vi "Call.vi"(6 "Error":errorcluster, 10 "PayloadCluster":T1 {"MetadataCluster"."AbsoluteTime" format="%<%x %.3X>T"}, 11 "Actor":refnum<class "Actor.lvclass">) -> (2 "PayloadCluster":T1 {"MetadataCluster"."AbsoluteTime" format="%<%x %.3X>T"}, 3 "Actor":refnum<class "Actor.lvclass">, 4 "Error":errorcluster)   [LabVIEW 2020, in "_Template.lvlib" / "{{Message}}.lvlib"]
uses:
  {{Message}}.lvlib
  Message/Message.lvclass
  jettl/jettl/jettl.lvlib
  jettl/jettl/Actor/Actor.lvclass
  jettl/jettl/LifecycleEnum.ctl
  jettl/jettl/TellOriginEnum.ctl
  jettl/jettl/MetadataCluster.ctl
  PayloadCluster.ctl
  jettl/jettl/CustomMetadata/CustomMetadata.lvclass
panel:
  # "This front panel should not be manipulated."
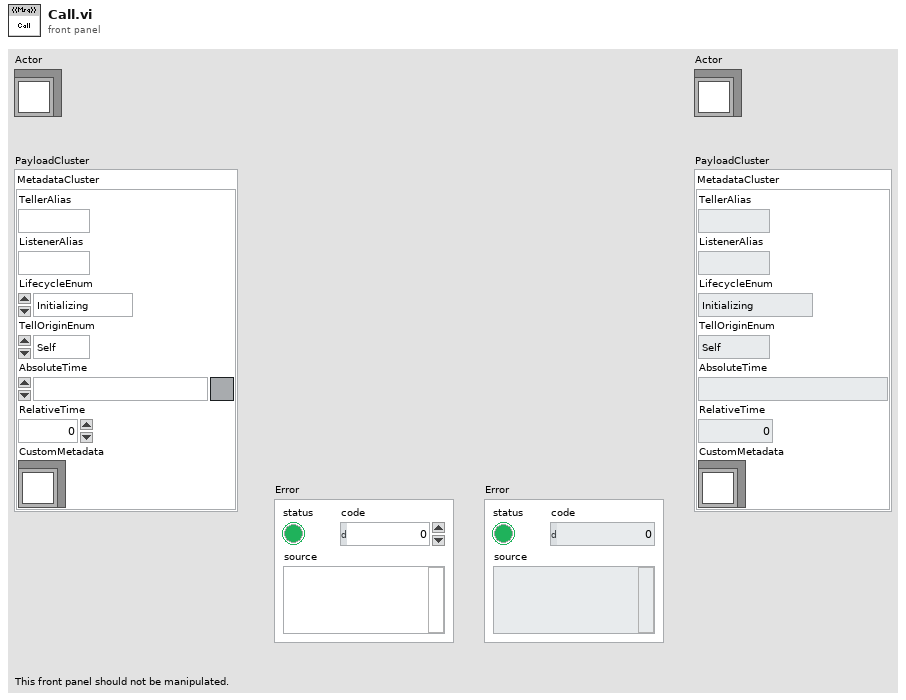
[diagram p1: front panel]
types:
  T1 = typedef "_Template.lvlib/{{Message}}.lvlib/PayloadCluster.ctl" = cluster{"MetadataCluster":T2}
  T2 = typedef "jettl.lvlib/MetadataCluster.ctl" = cluster{"TellerAlias":string, "ListenerAlias":string, "LifecycleEnum":T3, "TellOriginEnum":T4, "AbsoluteTime":timestamp, "RelativeTime":dbl, "CustomMetadata":refnum<class "CustomMetadata.lvclass">}
  T3 = typedef "jettl.lvlib/LifecycleEnum.ctl" = enum16{"Initializing", "SettingUp", "Starting", "Running", "Stopping", "TearingDown", "Terminated", "Abort"}
  T4 = typedef "jettl.lvlib/TellOriginEnum.ctl" = enum16{"Self", "Mediator", "Component"}
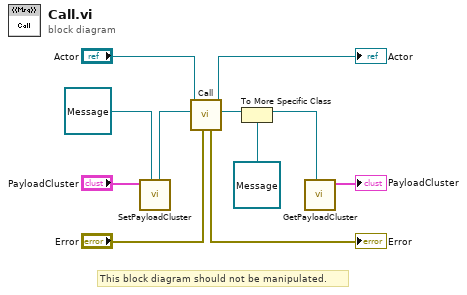
[diagram p0: block diagram]
diagram:
  # "This block diagram should not be manipulated."
  n1 = call "SetPayloadCluster.vi"("Message"=refnum<class "Message.lvclass"> refnum ("_Template.lvlib:MessageTemplate.lvlib:{{Name}}.lvlib:ConcreteMessage.lvclass"), "PayloadCluster"="PayloadCluster") -> ("Message"=w2:refnum<class "Message.lvclass">)  [unwired: 9 in]
  n2 = call "Call.vi"("Error"="Error", "Message"=w2, "Actor"="Actor") -> ("Message"=w6:refnum<class "Message.lvclass">, "Actor"=→"Actor":refnum<class "Actor.lvclass">, "Error"=→"Error":errorcluster)  [unwired: 6 in]
  n3 = To More Specific Class(target class=refnum<class "Message.lvclass"> refnum ("_Template.lvlib:Templates.lvlib:{{Name}}Message.lvlib:{{Name}}Message.lvclass"), reference=w6) -> (specific class reference=w5:refnum<class "Message.lvclass">)  [unwired: 1 in, 1 out]
  n4 = call "GetPayloadCluster.vi"("Message"=w5) -> ("PayloadCluster"=→"PayloadCluster":T1)  [unwired: 10 in]
